vi "Update Enum Mapper.vi"(8 "error in":errorcluster, 10 "RPC Message Name":string, 11 "VI in":refnum<vi>) -> (0 "error out":errorcluster)   [LabVIEW 2019, in "gRPC Template Creation Utility.lvlib"]
uses:
  gRPC Template Creation Utility.lvlib
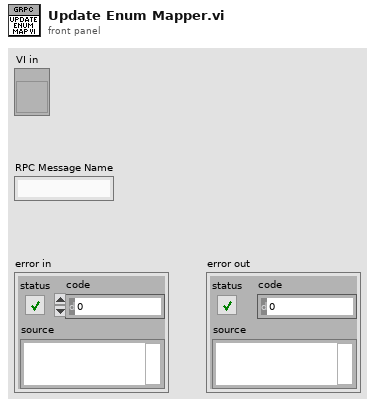
[diagram p1: front panel]
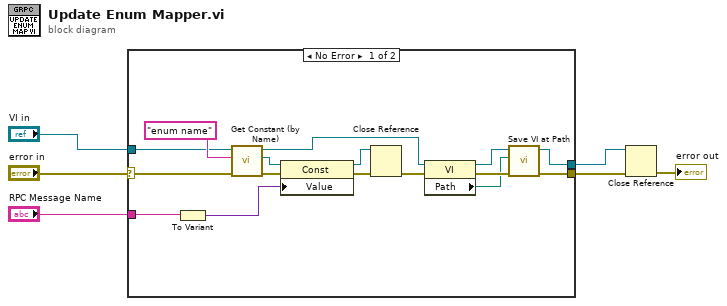
[diagram p0: block diagram]
diagram:
  n1 = case shown="No Error" "error in" {
    selector: "error in" -> [w14 w23]
    tunnel: [w8 w23] -> w2
    tunnel: [w10 w24] -> w3
    tunnel: "VI in" -> [w16 w24]
    tunnel: "RPC Message Name" -> [w15 _]
    frame No Error {
      n2 = To Variant(anything=w15) -> (Variant=w20:variant)
      n3 = call "Get Constant (by Name).vi"("error in (no error)"=w14, "Constant Label"="enum name" ("name/order"), "Owner VI in"=w16) -> ("error out"=w17:errorcluster, "Const ref out"=w19:refnum<vi>, "Owner VI out"=w12:refnum<vi>)  [unwired: 5 in, 1 out]
      n4 = property class="Const"(reference=w19, error in=w17, "Value"=w20) -> (reference out=w22:refnum<vi>, error out=w21:errorcluster)
      n5 = Close Reference(reference=w22, error in (no error)=w21) -> (error out=w13:errorcluster)
      n6 = property class="VI"(reference=w12, error in=w13) -> (reference out=w11:refnum<vi>, error out=w9:errorcluster, "Path"=w7:path)
      n7 = call "Save VI at Path.vi"("error in (no error)"=w9, "Path"=w7, "VI in"=w11) -> ("error out"=w8:errorcluster, "VI out"=w10:refnum<vi>)  [unwired: 6 in, 1 out]
    }
    frame Error {
    }
  }
  n8 = Close Reference(reference=w3, error in (no error)=w2) -> (error out=→"error out":errorcluster)
